vi "Check Reset.vi"(6 "Loop Data in":T1, 11 "Sequence in":refnum<class "Sequence.lvclass">) -> (4 "Loop Data":T1)   [LabVIEW 2023, in "VolatusSeq.lvlib" / "Sequence.lvclass"]
uses:
  Sequence.lvclass
  Loop Data.ctl
  Volatus/MessageQ/MessageQ.lvclass
  Sequence Time.ctl
  Sequence.lvclass/Sequence.ctl
  State/State.lvclass
  VolatusSeq.lvlib
  VolatusSeqConfig/Debug Flags.ctl
  VolatusSeqConfig/VolatusSeqConfig.lvlib
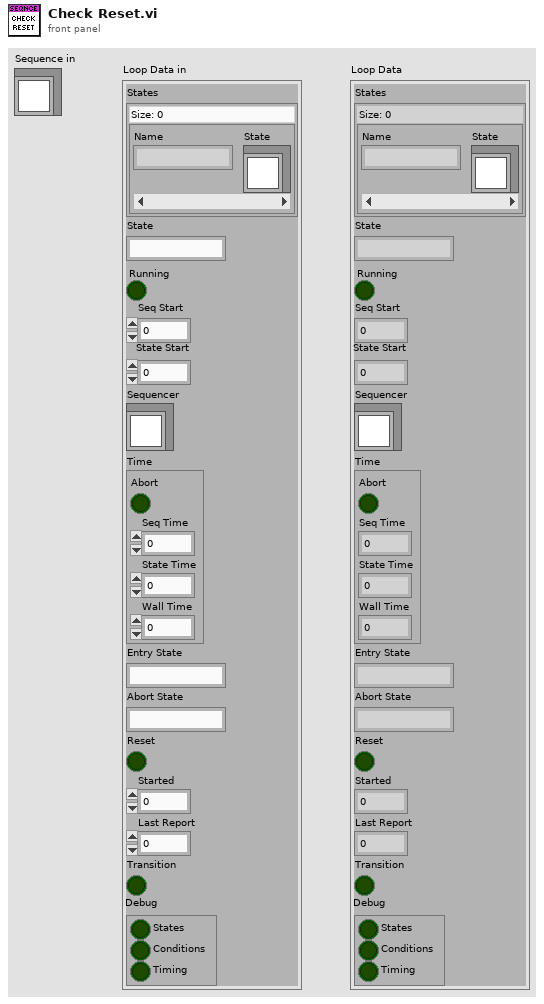
[diagram p1: front panel]
types:
  T1 = typedef "VolatusSeq.lvlib/Sequence.lvclass/Loop Data.ctl" = cluster{"States":map{string, refnum<class "State.lvclass">}, "State":string, "Running":bool, "Seq Start":dbl, "State Start":dbl, "Sequencer":refnum<class "MessageQ.lvclass">, "Time":T2, "Entry State":string, "Abort State":string, "Reset":bool, "Started":dbl, "Last Report":dbl, "Transition":bool, "Debug":T3}
  T2 = typedef "VolatusSeq.lvlib/Sequence Time.ctl" = cluster{"Abort":bool, "Seq Time":dbl, "State Time":dbl, "Wall Time":dbl}
  T3 = typedef "VolatusSeqConfig.lvlib/Debug Flags.ctl" = cluster{"States":bool, "Conditions":bool, "Timing":bool}
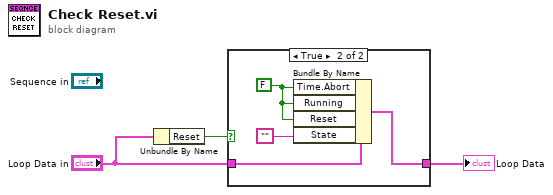
[diagram p0: block diagram]
diagram:
  n1 = Unbundle By Name("Loop Data in") -> ("Reset"=w1:bool)
  n2 = case shown="True" w1 {
    tunnel: "Loop Data in" -> [w4 w8]
    tunnel: [w4 w7] -> w3
    frame False {
    }
    frame True {
      w6 = FALSE ("Abort")
      n3 = Bundle By Name(cluster=w8, "Time.Abort"=w6, "Running"=w6, "Reset"=w6, "State"="") -> (w7:T1)
    }
  }
  "Loop Data" <- w3
